vi "getParent.vi"(8 "error in (no error)":errorcluster, 11 "TreeNode in":refnum<class "TreeNode.lvclass">) -> (0 "error out":errorcluster, 2 "Parent":refnum<data-value>, 3 "TreeNode out":refnum<class "TreeNode.lvclass">)   [LabVIEW 2014, in "Tree.lvlib" / "TreeNode.lvclass"]
doc: "Gets the parent nodes."
uses:
  <userlib>/AdvancedDataStructures/ClassBased/TreeNode/TreeNode.lvclass
  <userlib>/AdvancedDataStructures/ClassBased/TreeNode/TreeNode.lvclass/TreeNode.ctl
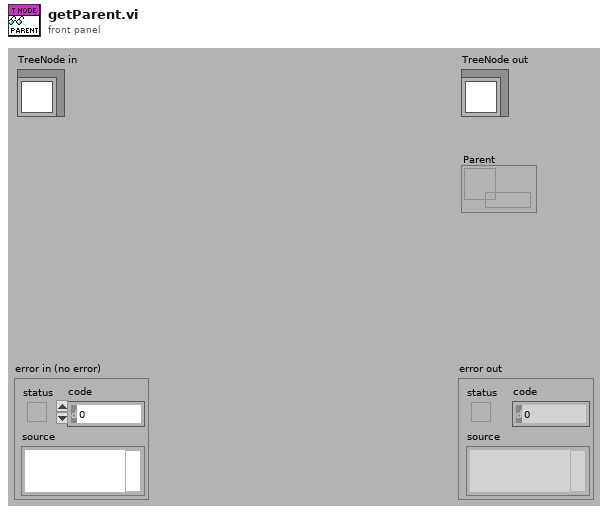
[diagram p1: front panel]
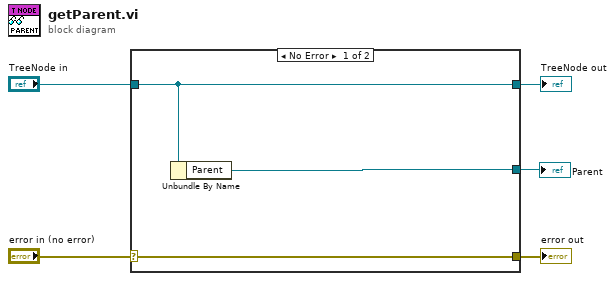
[diagram p0: block diagram]
diagram:
  n1 = case shown="No Error" "error in (no error)" {
    selector: "error in (no error)" -> [w8 w9]
    tunnel: [w8 w9] -> w4
    tunnel: [w6 w10] -> w3
    tunnel: "TreeNode in" -> [w6 w10]
    tunnel: [w7 _] -> w1
    frame No Error {
      n2 = Unbundle By Name(w6) -> ("Parent"=w7:refnum<data-value>)
    }
    frame Error {
    }
  }
  "error out" <- w4
  "TreeNode out" <- w3
  "Parent" <- w1
